vi "CmdStart.vi"(4 "error in (no error)":errorcluster caption="entrée d'erreur (pas d'erreur)", 6 "Path":string, 7 "Path":path=path "D:/WORK/SW/Embedded_SW_test/PROJECT/05/03/CFG_00") -> (0 "Error out":errorcluster)   [LabVIEW 2013]
panel:
  out "standard error":string caption="erreur standard"
  out "standard output":string caption="sortie standard"
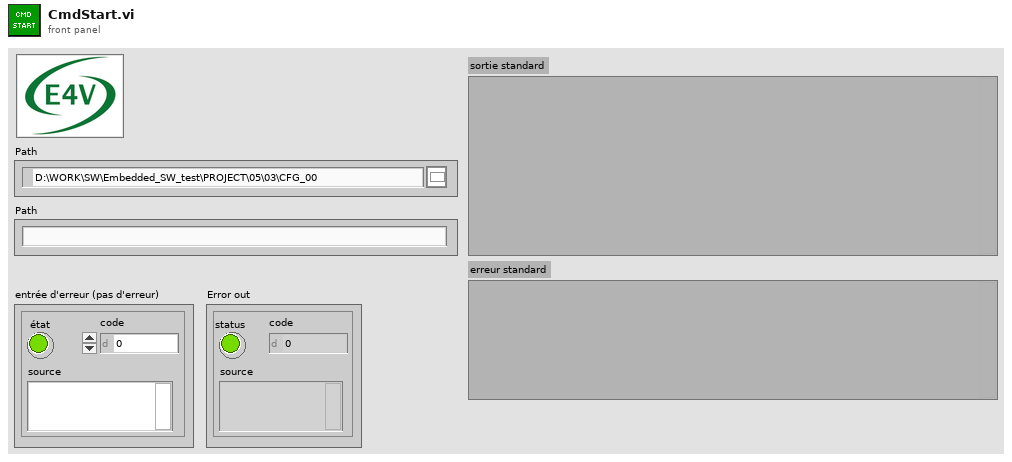
[diagram p1: front panel]
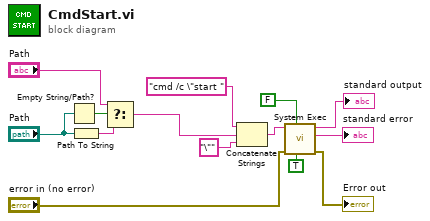
[diagram p0: block diagram]
diagram:
  n1 = Empty String/Path?(string/path="Path") -> (empty?=w4:bool)
  n2 = Path To String(path="Path") -> (string=w2:string)
  n3 = Select(t="Path", s=w4, f=w2) -> (s? t:f=w1:string)
  n4 = Concatenate Strings("cmd /c \"start " ("command line"), w1, "\"" ("chaîne")) -> (w9:string)
  n5 = call <vilib>:"System Exec.vi"("run minimized? (F)"=TRUE, "wait until completion? (T)"=FALSE, "error in (no error)"="error in (no error)", "command line"=w9) -> ("error out"=→"Error out":errorcluster, "standard error"=→"standard error":string, "standard output"=→"standard output":string)  [unwired: 4 in, 1 out]
